vi "retrieve_error_from_queue.vi"(8 "error in (no error)":errorcluster, 11 "ErrorController in":refnum<class "ErrorController.lvclass">) -> (0 "error out":errorcluster, 2 "error information":T1, 3 "ErrorController out":refnum<class "ErrorController.lvclass">)   [LabVIEW 2010, in "ErrorController.lvclass"]
uses:
  ErrorController.lvclass
  error_cluster.ctl
  ErrorController.lvclass/ErrorController.ctl
  BalloonNotifier/BalloonNotifier/BalloonNotifier.lvclass
  class_data.vi
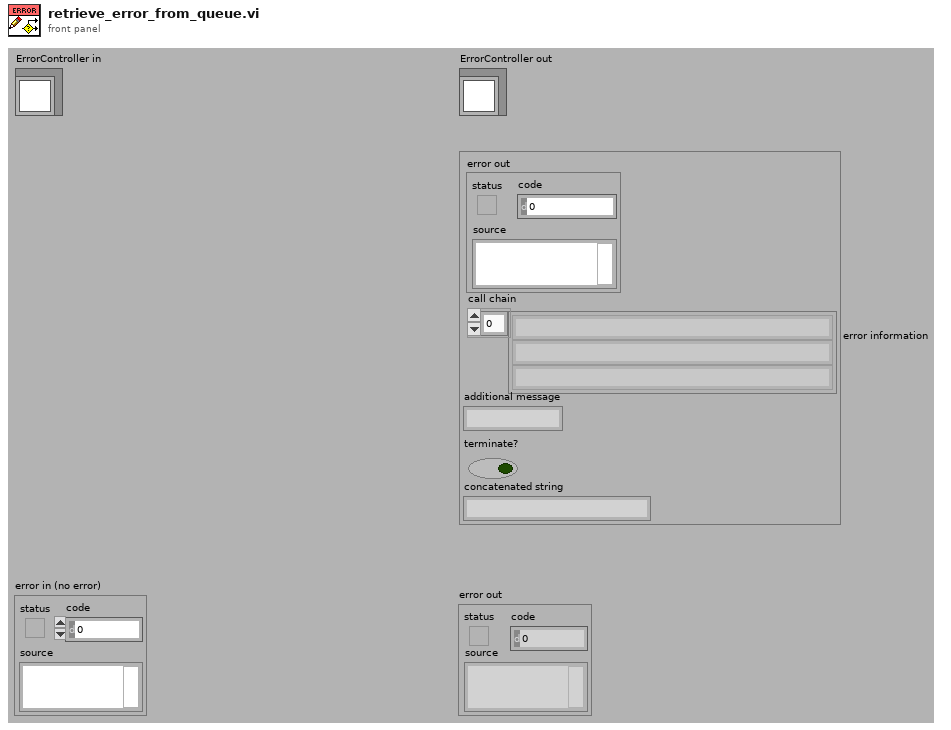
[diagram p1: front panel]
types:
  T1 = typedef "ErrorController.lvclass/error_cluster.ctl" = cluster{"error out":errorcluster, "call chain":string[], "additional message":string, "terminate?":bool, "concatenated string":string}
  T2 = typedef "ErrorController.lvclass/queue controller.ctl" = refnum<queue>
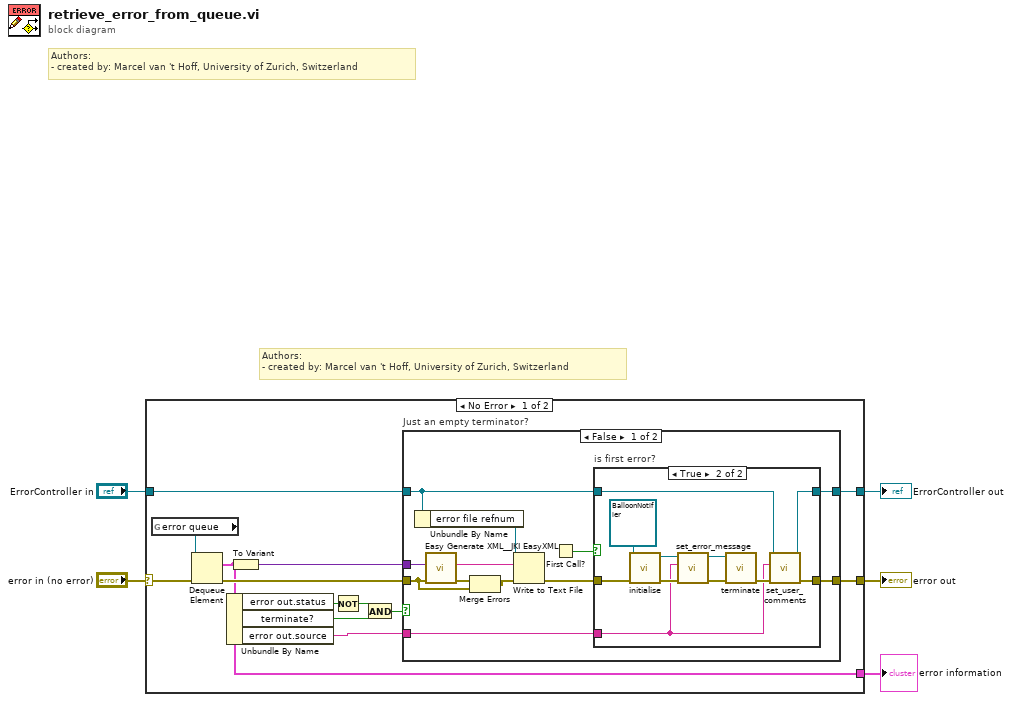
[diagram p0: block diagram]
diagram:
  # "Authors: \n- created by: Marcel van 't Hoff, University of Zurich, Switzerland"
  # "Authors: \n- created by: Marcel van 't Hoff, University of Zurich, Switzerland"
  n1 = case shown="No Error" "error in (no error)" {
    selector: "error in (no error)" -> [w17 w47]
    tunnel: [w7 w47] -> w4
    tunnel: [w6 w46] -> w2
    tunnel: "ErrorController in" -> [w15 w46]
    tunnel: [w13 _] -> w1
    frame No Error {
      n2 = global read "class_data.vi" "error queue"() -> (w18:T2)
      n3 = Dequeue Element(queue=w18, error in (no error)=w17) -> (element=w13:T1, error out=w16:errorcluster)  [unwired: 1 in, 2 out]
      n4 = Unbundle By Name(w13) -> ("error out.status"=w12:bool, "terminate?"=w11:bool, "error out.source"=w8:string)
      n5 = To Variant(anything=w13) -> (Variant=w14:variant)
      n6 = Not(x=w12) -> (.not. x?=w10:bool)
      n7 = And(x=w10, y=w11) -> (x .and. y?=w9:bool)
      n8 = case "Just an empty terminator?" shown="False" w9 {
        tunnel: w16 -> [w25 w44]
        tunnel: [w19 w44] -> w7
        tunnel: w15 -> [w24 w45]
        tunnel: w14 -> [w28 _]
        tunnel: [w23 w45] -> w6
        tunnel: w8 -> [w21 _]
        frame False {
          n9 = Unbundle By Name(w24) -> ("error file refnum"=w29:refnum<file>)
          n10 = call <vilib>:"Easy Generate XML__JKI EasyXML.vi"("error in (no error)"=w25, "LabVIEW Data"=w28) -> ("error out"=w30:errorcluster, "XML String"=w27:string)  [unwired: 8 in]
          n11 = Merge Errors(w30, w25) -> (w26:errorcluster)
          n12 = Write to Text File(file (use dialog)=w29, text=w27, error in=w26) -> (error out=w20:errorcluster)  [unwired: 1 in, 2 out]
          n13 = First Call?() -> (First Call?: T/F=w22:bool)
          n14 = case "is first error?" shown="True" w22 {
            tunnel: w20 -> [w31 w41]
            tunnel: [w31 w34] -> w19
            tunnel: w21 -> [_ w33]
            tunnel: w24 -> [w32 w37]
            tunnel: [w32 w36] -> w23
            frame False {
            }
            frame True {
              n15 = call-dynamic "initialise.vi"("error in (no error)"=w41, "BalloonNotifier in"=refnum<class "BalloonNotifier.lvclass"> refnum) -> ("error out"=w40:errorcluster, "BalloonNotifier out"=w42:refnum<class "BalloonNotifier.lvclass">)  [unwired: 8 in]
              n16 = call-dynamic "set_error_message.vi"("error in (no error)"=w40, "error message in"=w33, "BalloonNotifier in"=w42) -> ("error out"=w38:errorcluster, "BalloonNotifier out"=w39:refnum<class "BalloonNotifier.lvclass">)  [unwired: 7 in]
              n17 = call-dynamic "terminate.vi"("error in (no error)"=w38, "BalloonNotifier in"=w39) -> ("error out"=w35:errorcluster)  [unwired: 8 in, 1 out]
              n18 = call-dynamic "set_user_comments.vi"("error in (no error)"=w35, "details source"=w33, "ErrorController in"=w37) -> ("error out"=w34:errorcluster, "ErrorController out"=w36:refnum<class "ErrorController.lvclass">)  [unwired: 7 in]
            }
          }
        }
        frame True {
        }
      }
    }
    frame Error {
    }
  }
  "error out" <- w4
  "ErrorController out" <- w2
  "error information" <- w1
